vi "G#Debugger_RunVI.vi"(0 "vi reference":refnum<vi>, 2 "wait until done":bool, 5 "error in (no error)":errorcluster) -> (10 "class name":string, 12 "object ID":u32 format="%x", 15 "message":string, 16 "not a refnum?":bool, 19 "error out":errorcluster)   [LabVIEW 2020, in "G#Debugger.lvlib"]
doc: "Runs the VI selected in Active Debug."
uses:
  <vilib>/addons/_AddQ/G#Debugger/G#Debugger.lvlib
  <vilib>/addons/_AddQ/G#Object/G#Object.lvclass
panel:
  out "cached object out":refnum<class "G#Object.lvclass">
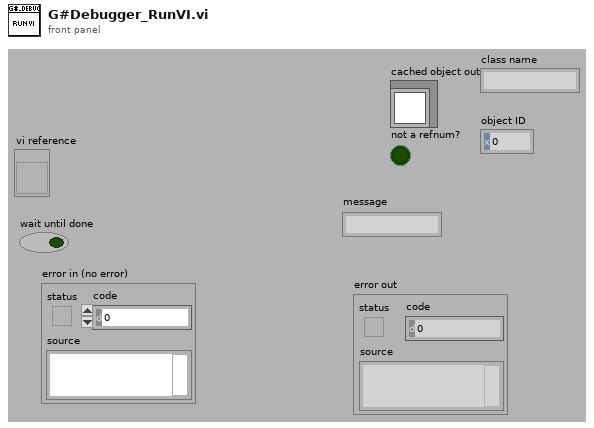
[diagram p1: front panel]
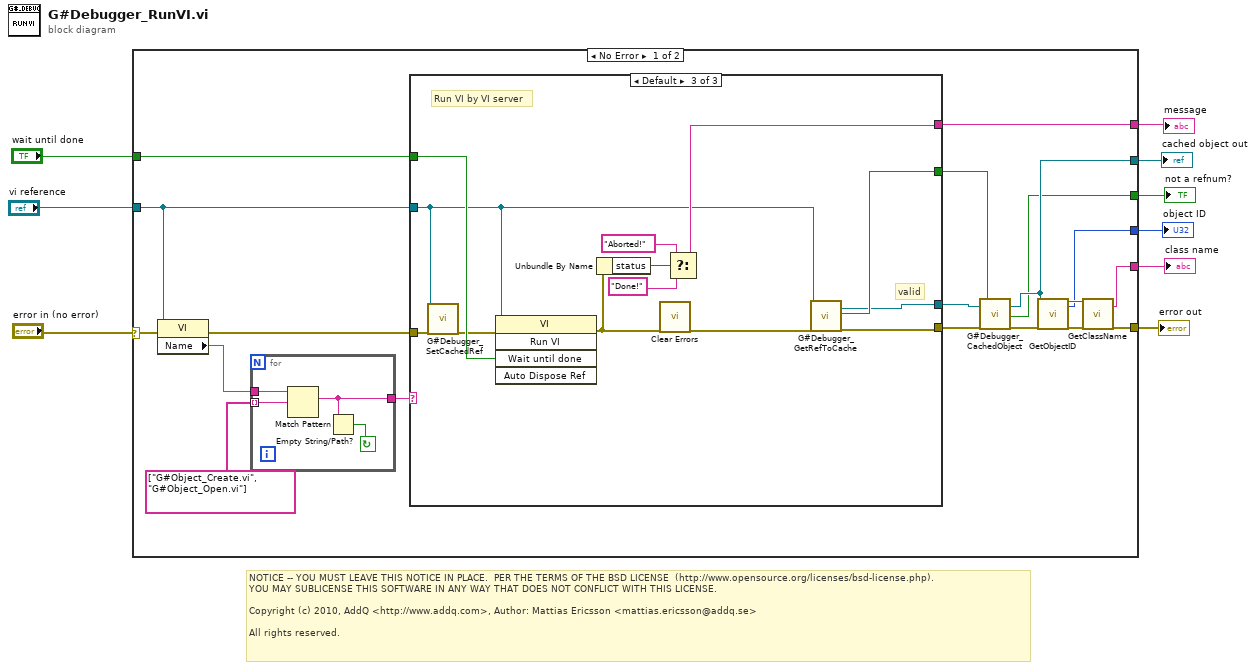
[diagram p0: block diagram]
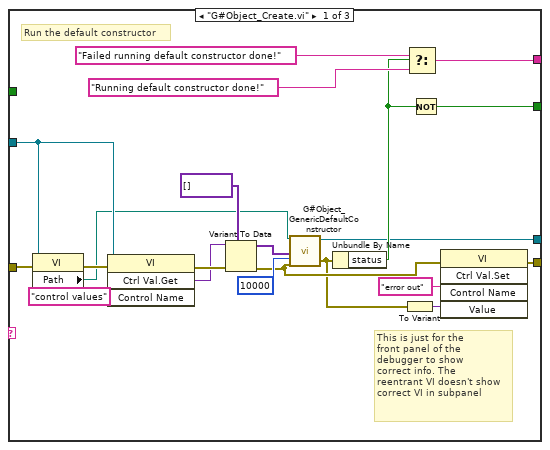
[diagram p2: hidden frame]
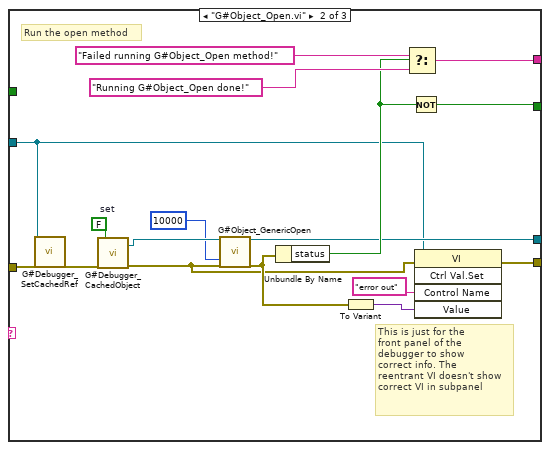
[diagram p3: hidden frame]
diagram:
  # "NOTICE -- YOU MUST LEAVE THIS NOTICE IN PLACE.  PER THE TERMS OF THE BSD LICENSE  (http://www.opensource.org/licenses/bsd-license.php).\nYOU MAY SUBLICENSE THIS SOFTWARE IN ANY WAY THAT DOES NOT CONFLICT WITH THIS LICENSE.\n\nCopyright (c) 2010, AddQ <http://www.addq.com>, Author: Mattias Ericsson <mattias.ericsson@addq.se>\n\nAll rights reserved."
  n1 = case shown="No Error" "error in (no error)" {
    selector: "error in (no error)" -> [w19 w84]
    tunnel: "wait until done" -> [w28 _]
    tunnel: [w27 _] -> w8
    tunnel: [w13 _] -> w7
    tunnel: [w15 _] -> w6
    tunnel: [w24 w84] -> w5
    tunnel: [w23 _] -> w4
    tunnel: [w22 _] -> w3
    tunnel: "vi reference" -> [w20 _]
    frame No Error {
      n2 = property class="VI"(reference=w20, error in=w19) -> (error out=w21:errorcluster, "Name"=w18:string)  [unwired: 1 out]
      n3 = for {
        tunnel: w18 -> [w32]
        tunnel: [w29] -> w11
        tunnel: string[] ["G#Object_Create.vi", "G#Object_Open.vi"] -> [w31] mode=indexing
        stop <- w30 continue-if-true
        n4 = Match Pattern(string=w32, regular expression=w31) -> (match substring=w29:string)  [unwired: 1 in, 3 out]
        n5 = Empty String/Path?(string/path=w29) -> (empty?=w30:bool)
      }
      n6 = case shown="Default" w11 {
        tunnel: w28 -> [_ _ w83]
        tunnel: [w44 w70 w81] -> w27
        tunnel: [w38 w66 w75] -> w12
        tunnel: [w37 w59 w73] -> w17
        tunnel: [w39 w63 w74] -> w14
        tunnel: w21 -> [w40 w58 w78]
        tunnel: w20 -> [w46 w56 w76]
        frame "G#Object_Create.vi" {
          # "This is just for the\nfront panel of the\ndebugger to show\ncorrect info. The\nreentrant VI doesn't show\ncorrect VI in subpanel"
          # "Run the default constructor"
          n7 = property class="VI"(reference=w46, error in=w40) -> (error out=w47:errorcluster, "Path"=w45:path)  [unwired: 1 out]
          n8 = invoke class="VI" method="Ctrl Val.Get"(reference=w46, error in=w47, "Control Name"="control values") -> (error out=w51:errorcluster, "Get Control Value Variant"=w50:variant)  [unwired: 1 in, 2 out]
          n9 = Variant To Data(error in=w51, type=variant[] [], Variant=w50) -> (data=w49:variant[], error out=w36:errorcluster)
          n10 = call <vilib>:"G#Object_GenericDefaultConstructor.vi"("class path"=w45, "control values"=w49, "timeout in ms (-1)"=10000 ("timeout (ms)"), "error in (no error)"=w36) -> ("reference out"=w39:refnum<class "G#Object.lvclass">, "error out"=w33:errorcluster)  [unwired: 13 in, 1 out]
          n11 = Unbundle By Name(w33) -> ("status"=w41:bool)
          n12 = To Variant(anything=w33) -> (Variant=w34:variant)
          n13 = Select(t="Failed running default constructor done!", s=w41, f="Running default constructor done!") -> (s? t:f=w44:string)
          n14 = Not(x=w41) -> (.not. x?=w38:bool)
          n15 = invoke class="VI" method="Ctrl Val.Set"(error in=w36, "Control Name"="error out", "Value"=w34) -> (error out=w37:errorcluster)  [unwired: 2 in, 4 out]
        }
        frame "G#Object_Open.vi" {
          w65 = FALSE  # set
          # "This is just for the\nfront panel of the\ndebugger to show\ncorrect info. The\nreentrant VI doesn't show\ncorrect VI in subpanel"
          # "Run the open method"
          n16 = call <vilib>:"G#Debugger_SetCachedRef.vi"("MethodVIref"=w56, "error in (no error)"=w58) -> ("error out"=w57:errorcluster)  [unwired: 17 in]
          n17 = call <vilib>:"G#Debugger_CachedObject.vi"("error in (no error)"=w57, "set"=w65) -> ("cached object out"=w64:refnum<class "G#Object.lvclass">, "error out"=w55:errorcluster)  [unwired: 15 in, 1 out]
          n18 = call-dynamic "G#Object_GenericOpen.vi"("reference in"=w64, "timeout in ms (-1)"=10000 ("timeout (ms)"), "error in (no error)"=w55) -> ("reference out"=w63:refnum<class "G#Object.lvclass">, "error out"=w60:errorcluster)  [unwired: 14 in, 1 out]
          n19 = Unbundle By Name(w60) -> ("status"=w67:bool)
          n20 = To Variant(anything=w60) -> (Variant=w54:variant)
          n21 = Select(t="Failed running G#Object_Open method!", s=w67, f="Running G#Object_Open done!") -> (s? t:f=w70:string)
          n22 = Not(x=w67) -> (.not. x?=w66:bool)
          n23 = invoke class="VI" method="Ctrl Val.Set"(reference=w56, error in=w55, "Control Name"="error out", "Value"=w54) -> (error out=w59:errorcluster)  [unwired: 1 in, 4 out]
        }
        frame Default {
          # "valid"
          # "Run VI by VI server"
          n24 = call <vilib>:"G#Debugger_SetCachedRef.vi"("MethodVIref"=w76, "error in (no error)"=w78) -> ("error out"=w77:errorcluster)  [unwired: 17 in]
          n25 = invoke class="VI" method="Run VI"(reference=w76, error in=w77, "Wait until done"=w83) -> (error out=w72:errorcluster)  [unwired: 2 in, 4 out]
          n26 = Unbundle By Name(w72) -> ("status"=w82:bool)
          n27 = call <vilib>:"Clear Errors.vi"("error in (no error)"=w72) -> ("error out"=w71:errorcluster)  [unwired: 5 in, 1 out]
          n28 = Select(t="Aborted!", s=w82, f="Done!") -> (s? t:f=w81:string)
          n29 = call <vilib>:"G#Debugger_GetRefToCache.vi"("MethodVIref"=w76, "error in (no error)"=w71) -> ("cached object out"=w74:refnum<class "G#Object.lvclass">, "valid"=w75:bool, "error out"=w73:errorcluster)  [unwired: 15 in]
        }
      }
      n30 = call <vilib>:"G#Debugger_CachedObject.vi"("cached object"=w14, "error in (no error)"=w17, "set"=w12) -> ("cached object out"=w15:refnum<class "G#Object.lvclass">, "not a refnum?"=w13:bool, "error out"=w16:errorcluster)  [unwired: 14 in]
      n31 = call-dynamic "GetObjectID.vi"("reference in"=w15, "error in (no error)"=w16) -> ("reference out"=w26:refnum<class "G#Object.lvclass">, "object ID"=w22:u32, "error out"=w25:errorcluster)  [unwired: 15 in]
      n32 = call-dynamic "GetClassName.vi"("reference in"=w26, "error in (no error)"=w25) -> ("class name"=w23:string, "error out"=w24:errorcluster)  [unwired: 13 in, 3 out]
    }
    frame Error {
    }
  }
  "error out" <- w5
  "message" <- w8
  "cached object out" <- w6
  "not a refnum?" <- w7
  "class name" <- w4
  "object ID" <- w3
